vi "Solartron 1260 multifile freq scan feb 16.vi"() -> ()   [LabVIEW 2014]
doc: "This VI configures and reads back a single measurement. \n\nNote:\nYou might need to extend the timeout set in the Wait Conditions subVI."
uses:
  <vilib>/Analysis/baseanly.llb/Mean (DBL).vi
  <vilib>/Utility/file.llb/Write To Spreadsheet File (DBL).vi
  <vilib>/Utility/file.llb/Write To Spreadsheet File (string).vi
  <instrlib>/Solartron 1260/Solartron 1260.lvlib
  <vilib>/Analysis/NI_AALBase.lvlib
panel:
  out "Current spectrum":dbl
  out "Current point":dbl
  out "XY Graph 2":cluster{dbl[], dbl[]}[](graph)
  in  "Measurement 2":T1 {"Result Type(0: [Z, Theta] for: Z1 or Z2)" items=["[Z, Theta]       for: Z1 or Z2", "[Y, Theta]       for: Y1 or Y2", "[r, Theta]        for: Fnc( ), V1, V2, V1/V2, V2/V1 or I", "[r(dB), Theta]  for: Fnc( ), V1, V2, V1/V2 or V2/V1", "[r, t]                 for: Fnc( ), V1, V2, V1/V2 or V2/V1", "[r (dB), t]          for: Fnc( ), V1, V2, V1/V2 or V2/V1", "[L(or C), R]      for: Z1, Y1, Z2, Y2 or Fnc( )", "[L(or C), Q]      for: Z1, Y1, Z2, Y2 or Fnc( )", "[L(or C), D]      for: Z1, Y1, Z2, Y2 or Fnc( ) ", "[R, X]              for: Z1 or Z2", "[G, B]              for: Y1 or Y2", "[a, b]               for: Fnc( ), V1, V2, V1/V2, V2/V1 or I"]; "Circuit (3:Parallel C, R)" items=["Serial L, R", "Serial C, R", "Parallel L, R", "Parallel C, R", "Auto"]; "Result Source(0:Z1 = V1/I)" items=["Z1 = V1/I", "Y1 = I/V1", "Z2 = V2/I", "Y2 = I/V2", "Function (  )", "V1", "V2", "V1/V2", "V2/V1", " I"]; "Variable (0:Frequency)" items=["Frequency", "Amplitude", "Baise"]}
  in  "Cluster":cluster{"DC bias (V)":dbl, "Amplitude (V)":dbl}={"DC bias (V)"=3.0, "Amplitude (V)"=3.0}
  out "File path":path
  out "XY Graph":cluster{dbl[], dbl[]}[](graph)
  in  "Measurement 1":T1 {"Result Type(0: [Z, Theta] for: Z1 or Z2)" items=["[Z, Theta]       for: Z1 or Z2", "[Y, Theta]       for: Y1 or Y2", "[r, Theta]        for: Fnc( ), V1, V2, V1/V2, V2/V1 or I", "[r(dB), Theta]  for: Fnc( ), V1, V2, V1/V2 or V2/V1", "[r, t]                 for: Fnc( ), V1, V2, V1/V2 or V2/V1", "[r (dB), t]          for: Fnc( ), V1, V2, V1/V2 or V2/V1", "[L(or C), R]      for: Z1, Y1, Z2, Y2 or Fnc( )", "[L(or C), Q]      for: Z1, Y1, Z2, Y2 or Fnc( )", "[L(or C), D]      for: Z1, Y1, Z2, Y2 or Fnc( ) ", "[R, X]              for: Z1 or Z2", "[G, B]              for: Y1 or Y2", "[a, b]               for: Fnc( ), V1, V2, V1/V2, V2/V1 or I"]; "Circuit (3:Parallel C, R)" items=["Serial L, R", "Serial C, R", "Parallel L, R", "Parallel C, R", "Auto"]; "Result Source(0:Z1 = V1/I)" items=["Z1 = V1/I", "Y1 = I/V1", "Z2 = V2/I", "Y2 = I/V2", "Function (  )", "V1", "V2", "V1/V2", "V2/V1", " I"]; "Variable (0:Frequency)" items=["Frequency", "Amplitude", "Baise"]}
  in  "measure spectra":bool
  out "Total scan time (hrs)":dbl
  out "Spectrum scan time (min)":dbl
  out "Freq. resolution (Hz)":dbl
  in  "Frequency options":T2={"End freq (Hz)"=0.0, "Start freq (Hz)"=0.0, "# of points in each spectrum"=0.0, "# of steps to average"=3.0, "# of spectra to measure"=3.0} {"Start freq (Hz)" format="%#_8f"; "End freq (Hz)" format="%#_8f"}
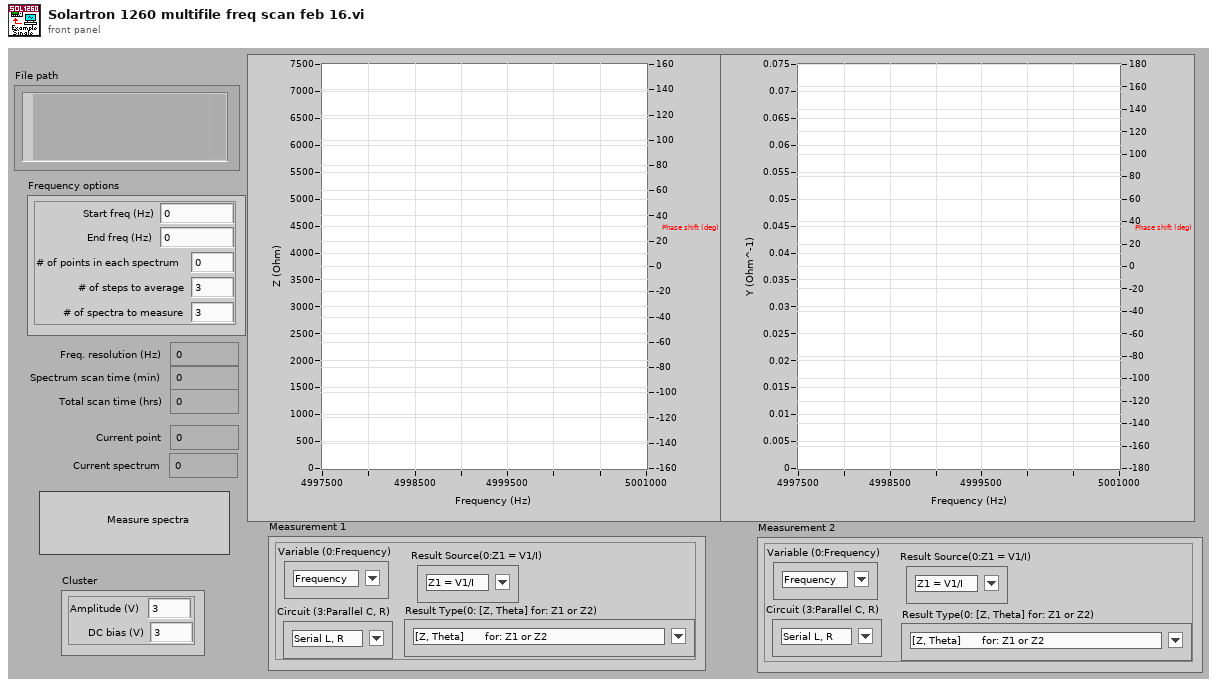
[diagram p1: front panel]
types:
  T1 = cluster{"Variable (0:Frequency)":u16, "Result Source(0:Z1 = V1/I)":u16, "Circuit (3:Parallel C, R)":u16, "Result Type(0: [Z, Theta] for: Z1 or Z2)":u16}
  T2 = cluster{"End freq (Hz)":dbl, "Start freq (Hz)":dbl, "# of points in each spectrum":dbl, "# of steps to average":dbl, "# of spectra to measure":dbl}
  T3 = enum16{"Off", "All", "Fail", "Pass", "Dump", "Dump all", "Plotter"}
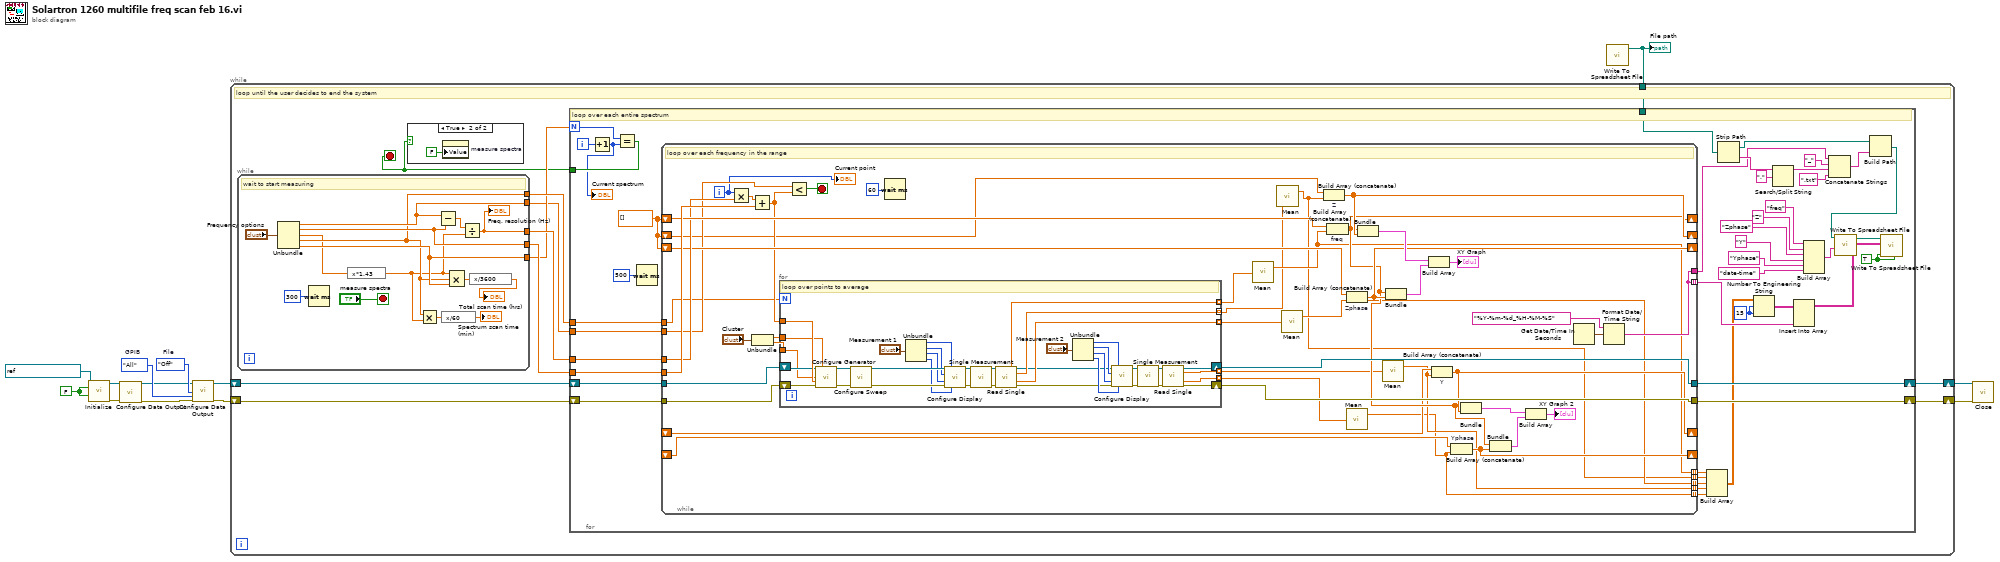
[diagram p0: block diagram]
diagram:
  w5 = T3."All"  # GPIB
  w6 = enum16{"Off", "All", "Fail", "Pass"}."Off"  # File
  w11 = FALSE ("ID Query (T: Check)")
  n1 = call <instrlib>:"Initialize.vi"("VISA resource name"=refnum<visa-resource-name> "GPIB2::4::INSTR", "ID Query (T: Check)"=w11, "Reset (T: Reset)"=w11) -> ("VISA resource name out"=w8:refnum<visa-resource-name>, "error out"=w9:errorcluster)  [unwired: 11 in]
  n2 = call <instrlib>:"Configure Data Output.vi"("VISA resource name"=w8, "error in (no error)"=w9) -> ("VISA resource name out"=w4:refnum<visa-resource-name>, "error out"=w2:errorcluster)  [unwired: 12 in]
  n3 = call <instrlib>:"Configure Data Output.vi"("VISA resource name"=w4, "File (1:All)"=w6, "GPIB (1:All)"=w5, "error in (no error)"=w2) -> ("VISA resource name out"=w3:refnum<visa-resource-name>, "error out"=w1:errorcluster)  [unwired: 10 in]
  n4 = call-poly <vilib>:"Write To Spreadsheet File.vi"() -> ("new file path (Not A Path if cancelled)"=w7:path)  [unwired: 8 in]
  "File path" <- w7
  n5 = while {
    shift-right: [w23] -> w12
    shift-left: w3 -> [w22]
    shift-right: [w24] -> w13
    shift-left: w1 -> [w21]
    tunnel: w7 -> [w17]
    stop <- w14 stop-if-true
    # "loop until the user decides to end the system"
    n6 = while {
      tunnel: [w39] -> w20
      tunnel: [w32] -> w19
      tunnel: [w38] -> w18
      tunnel: [w33] -> w16
      tunnel: [w35] -> w15
      stop <- "measure spectra" stop-if-true
      # "wait to start measuring"
      n7 = Unbundle("Frequency options") -> ("End freq (Hz)"=w35:dbl, "Start freq (Hz)"=w39:dbl, "# of points in each spectrum"=w26:dbl, "# of steps to average"=w32:dbl, "# of spectra to measure"=w33:dbl)
      n8 = Wait (ms)(milliseconds to wait=300) -> ()  [unwired: 1 out]
      n9 = expression code="x*1.43"(w26) -> (w27:dbl)
      n10 = Multiply(x=w32, y=w27) -> (x*y=w31:dbl)
      n11 = Subtract(x=w35, y=w39) -> (x-y=w40:dbl)
      n12 = expression code="x/60"(w31) -> (→"Spectrum scan time (min)":dbl)
      n13 = Compound Arithmetic op=MULTIPLY(w27, w32, w33) -> (w29:dbl)
      n14 = Divide(x=w40, y=w27) -> (x/y=w38:dbl)
      "Freq. resolution (Hz)" <- w38
      n15 = expression code="x/3600"(w29) -> (→"Total scan time (hrs)":dbl)
    }
    n16 = for {
      N: w16 -> [w56]
      tunnel: w20 -> [w79]
      tunnel: w15 -> [w78]
      tunnel: w19 -> [w77]
      tunnel: w18 -> [w76]
      tunnel: w17 -> [w65]
      shift-right: [w82] -> w23
      shift-left: w22 -> [w81]
      shift-right: [w83] -> w24
      shift-left: w21 -> [w80]
      tunnel: [w55] -> w14
      i -> [w54]
      w73 = TRUE ("append to file? (new file:F)")
      w74 = i16 15 ("precision (6)")
      w75 = dbl[] []
      # "loop over each entire spectrum"
      n17 = Increment(x=w54) -> (x+1=w41:i32)
      "Current spectrum" <- w41
      n18 = Equal?(x=w56, y=w41) -> (x = y?=w55:bool)
      n19 = Wait (ms)(milliseconds to wait=u32 500) -> ()  [unwired: 1 out]
      n20 = while {
        tunnel: [w124] -> w83
        tunnel: [w123] -> w82
        tunnel: w81 -> [w126]
        tunnel: w80 -> [w125]
        tunnel: w79 -> [w127]
        shift-right: [w101] -> _
        shift-left: w75 -> [w122]
        shift-right: [w115] -> _
        shift-left: w75 -> [w90]
        tunnel: w76 -> [w121]
        shift-right: [w117] -> _
        shift-left: w75 -> [w118]
        tunnel: [w88] -> w72 mode=indexing
        tunnel: [w86] -> w70 mode=indexing
        tunnel: [w87] -> w71 mode=indexing
        tunnel: w78 -> [w114]
        tunnel: w77 -> [w100]
        tunnel: [w111] -> w68 mode=indexing
        tunnel: [w111] -> w58
        shift-right: [w102] -> _
        shift-left: _ -> [w98]
        shift-right: [w99] -> _
        shift-left: _ -> [w97]
        tunnel: [w94] -> w43 mode=indexing
        tunnel: [w92] -> w42 mode=indexing
        i -> [w84]
        stop <- w109 stop-if-true
        # "loop over each frequency in the range"
        n21 = Multiply(x=w84, y=w121) -> (x*y=w96:dbl)
        n22 = Add(x=w96, y=w127) -> (x+y=w113:dbl)
        n23 = Unbundle("Cluster") -> ("DC bias (V)"=w107:dbl, "Amplitude (V)"=w106:dbl)
        n24 = for {
          N: w100 -> [_]
          tunnel: [w151] -> w89 mode=indexing
          tunnel: [w150] -> w85 mode=indexing
          tunnel: [w149] -> w91 mode=indexing
          tunnel: w113 -> [w148]
          shift-right: [w132] -> w123
          shift-left: w126 -> [w147]
          shift-right: [w131] -> w124
          shift-left: w125 -> [w146]
          tunnel: w107 -> [w145]
          tunnel: w106 -> [w144]
          tunnel: [w130] -> w95 mode=indexing
          tunnel: [w129] -> w93 mode=indexing
          # "loop over points to average"
          n25 = call <instrlib>:"Configure Generator.vi"("VISA resource name"=w147, "Voltage Bias(0.0 V)"=w145, "Voltage Amplitude(1.0 V)"=w144, "Frequency(1.0 Hz)"=w148, "error in (no error)"=w146) -> ("VISA resource name out"=w164:refnum<visa-resource-name>, "error out"=w163:errorcluster)  [unwired: 9 in]
          n26 = call <instrlib>:"Configure Sweep.vi"("VISA resource name"=w164, "error in (no error)"=w163) -> ("VISA resource name out"=w161:refnum<visa-resource-name>, "error out"=w162:errorcluster)  [unwired: 12 in]
          n27 = Unbundle("Measurement 1") -> ("Variable (0:Frequency)"=w155:u16, "Result Source(0:Z1 = V1/I)"=w153:u16, "Circuit (3:Parallel C, R)"=w154:u16, "Result Type(0: [Z, Theta] for: Z1 or Z2)"=w152:u16)
          n28 = call <instrlib>:"Configure Display.vi"("VISA resource name"=w161, "Variable (0:Frequency)"=w155, "Result Source(0:Z1 = V1/I)"=w153, "Circuit (3:Parallel C, R)"=w154, "error in (no error)"=w162, "Result Type(0: [Z, Theta] for: Z1 or Z2)"=w152) -> ("VISA resource name out"=w160:refnum<visa-resource-name>, "error out"=w159:errorcluster)  [unwired: 8 in]
          n29 = call <instrlib>:"Single Measurement.vi"("VISA resource name"=w160, "error in (no error)"=w159) -> ("VISA resource name out"=w157:refnum<visa-resource-name>, "error out"=w158:errorcluster)  [unwired: 12 in]
          n30 = call <instrlib>:"Read Single.vi"("VISA resource name"=w157, "error in (no error)"=w158) -> ("Variable"=w151:dbl, "VISA resource name out"=w133:refnum<visa-resource-name>, "Parameter 1"=w150:dbl, "Parameter2"=w149:dbl, "error out"=w134:errorcluster)  [unwired: 7 in, 2 out]
          n31 = Unbundle("Measurement 2") -> ("Variable (0:Frequency)"=w140:u16, "Result Source(0:Z1 = V1/I)"=w142:u16, "Circuit (3:Parallel C, R)"=w141:u16, "Result Type(0: [Z, Theta] for: Z1 or Z2)"=w143:u16)
          n32 = call <instrlib>:"Configure Display.vi"("VISA resource name"=w133, "Variable (0:Frequency)"=w140, "Result Source(0:Z1 = V1/I)"=w142, "Circuit (3:Parallel C, R)"=w141, "error in (no error)"=w134, "Result Type(0: [Z, Theta] for: Z1 or Z2)"=w143) -> ("VISA resource name out"=w135:refnum<visa-resource-name>, "error out"=w136:errorcluster)  [unwired: 8 in]
          n33 = call <instrlib>:"Single Measurement.vi"("VISA resource name"=w135, "error in (no error)"=w136) -> ("VISA resource name out"=w138:refnum<visa-resource-name>, "error out"=w137:errorcluster)  [unwired: 12 in]
          n34 = call <instrlib>:"Read Single.vi"("VISA resource name"=w138, "error in (no error)"=w137) -> ("VISA resource name out"=w132:refnum<visa-resource-name>, "Parameter 1"=w130:dbl, "Parameter2"=w129:dbl, "error out"=w131:errorcluster)  [unwired: 7 in, 3 out]
        }
        n35 = Less?(x=w114, y=w113) -> (x < y?=w109:bool)
        n36 = Wait (ms)(milliseconds to wait=u32 60) -> ()  [unwired: 1 out]
        n37 = call-poly <vilib>:"Mean.vi"("X"=w89) -> ("mean"=w88:dbl)  [unwired: 1 out]
        n38 = call-poly <vilib>:"Mean.vi"("X"=w85) -> ("mean"=w86:dbl)  [unwired: 1 out]
        n39 = call-poly <vilib>:"Mean.vi"("X"=w91) -> ("mean"=w87:dbl)  [unwired: 1 out]
        n40 = Build Array (concatenate) "Z"(w90, w86) -> (w115:dbl[])
        n41 = Build Array (concatenate) "freq"(w122, w88) -> (w101:dbl[])
        n42 = Build Array (concatenate) "Zphase"(w118, w87) -> (w117:dbl[])
        n43 = call-poly <vilib>:"Mean.vi"("X"=w93) -> ("mean"=w92:dbl)  [unwired: 1 out]
        n44 = Bundle(w101, w115) -> (w120:cluster{dbl[], dbl[]})  [unwired: 1 in]
        n45 = call-poly <vilib>:"Mean.vi"("X"=w95) -> ("mean"=w94:dbl)  [unwired: 1 out]
        n46 = Bundle(w101, w117) -> (w119:cluster{dbl[], dbl[]})  [unwired: 1 in]
        n47 = Build Array(w120, w119) -> (→"XY Graph":cluster{dbl[], dbl[]}[])
        n48 = Build Array (concatenate) "Y"(w98, w94) -> (w102:dbl[])
        n49 = Build Array (concatenate) "Yphase"(w97, w92) -> (w99:dbl[])
        n50 = Bundle(w101, w102) -> (w103:cluster{dbl[], dbl[]})  [unwired: 1 in]
        n51 = Bundle(w101, w99) -> (w104:cluster{dbl[], dbl[]})  [unwired: 1 in]
        n52 = Build Array(w103, w104) -> (→"XY Graph 2":cluster{dbl[], dbl[]}[])
        n53 = Get Date/Time In Seconds() -> (seconds since 1Jan1904=w112:timestamp)
        n54 = Format Date/Time String(time format string (%c)="%Y-%m-%d_%H-%M-%S", seconds (now)=w112) -> (date/time string=w111:string)  [unwired: 1 in]
        "Current point" <- w84
      }
      n55 = Build Array(w72, w70, w71, w43, w42) -> (w67:dbl[][])
      n56 = Strip Path(path=w65) -> (stripped path=w57:path, name=w60:string)
      n57 = Number To Engineering String(2:w74, 3:w74, 4:w67) -> (0:w69:string[][])  [unwired: 1 in]
      n58 = Search/Split String(string=w60, search string/char (-)=".") -> (substring before match=w61:string)  [unwired: 1 in, 2 out]
      n59 = Insert Into Array(array=w69, new element=w68) -> (w66:string[][])  [unwired: 2 in]
      n60 = Build Array("freq", "Z", "Zphase", "Y", "Yphase", "date-time") -> (w50:string[])
      n61 = Concatenate Strings(w58, "_" ("string"), w61, ".txt" ("string")) -> (w63:string)
      n62 = Build Path(base path=w57, name or relative path=w63) -> (appended path=w49:path)
      n63 = call-poly <vilib>:"Write To Spreadsheet File.vi"("1D data"=w50, "file path (dialog if empty)"=w49) -> ("new file path (Not A Path if cancelled)"=w48:path)  [unwired: 6 in]
      n64 = call-poly <vilib>:"Write To Spreadsheet File.vi"("transpose? (no:F)"=w73, "append to file? (new file:F)"=w73, "2D data"=w66, "file path (dialog if empty)"=w48) -> ()  [unwired: 4 in, 1 out]
    }
    n65 = case shown="True" w14 {
      frame False {
      }
      frame True {
        n66 = property on="measure spectra" class="Bool (strict)"("Value"=FALSE ("measure spectrum")) -> ()  [unwired: 2 in, 2 out]
      }
    }
  }
  n67 = call <instrlib>:"Close.vi"("VISA resource name"=w12, "error in (no error)"=w13) -> ()  [unwired: 13 in, 1 out]
